vi "02read_data_conection.vi"(0 "IP":string, 1 "bytes to read":u8, 2 "Puerto":u16, 3 "Time Out":u16, 4 "string to write":string="ÿ\u0003") -> (5 "data out":string, 6 "error out":errorcluster)   [LabVIEW 2010]
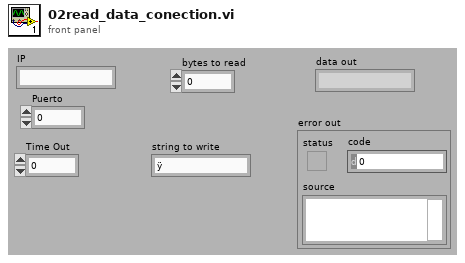
[diagram p1: front panel]
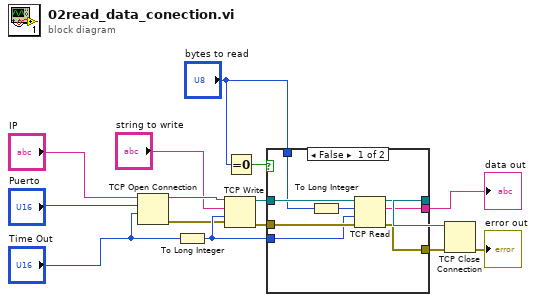
[diagram p0: block diagram]
diagram:
  n1 = TCP Open Connection(address="IP", remote port or service name="Puerto", timeout ms (60000)="Time Out") -> (connection ID=w12:refnum<k5>, error out=w1:errorcluster)  [unwired: 2 in]
  n2 = To Long Integer(number="Time Out") -> (32bit integer=w9:i32)
  n3 = TCP Write(connection ID=w12, data in="string to write", error in (no error)=w1, 9:w9) -> (connection ID out=w6:refnum<k5>, error out=w8:errorcluster)  [unwired: 1 out]
  n4 = Equal To 0?(x="bytes to read") -> (x = 0?=w3:bool)
  n5 = case shown="False" w3 {
    tunnel: [w23 w24] -> w11
    tunnel: [w22 w25] -> w10
    tunnel: w9 -> [w16 _]
    tunnel: w8 -> [w20 w24]
    tunnel: w6 -> [w19 w25]
    tunnel: "bytes to read" -> [w18 _]
    tunnel: [w17 _] -> w5
    frame False {
      n6 = To Long Integer(number=w18) -> (32bit integer=w21:i32)
      n7 = TCP Read(connection ID=w19, bytes to read=w21, error in (no error)=w20, 9:w16) -> (connection ID out=w22:refnum<k5>, data out=w17:string, error out=w23:errorcluster)  [unwired: 1 out]
    }
    frame True {
    }
  }
  "data out" <- w5
  n8 = TCP Close Connection(connection ID=w10, error in (no error)=w11) -> (error out=→"error out":errorcluster)  [unwired: 1 in, 1 out]
